vi "SupportedHardware.vi"() -> (3 "Supported Hardware":string[](array[string]))   [LabVIEW 2017, in "McsaFpgaAcquisition.lvlib"]
uses:
  <vilib>/addons/InsightCM/Devices/Shared/Mcsa/McsaFpgaAcquisition/McsaFpgaAcquisition.lvlib
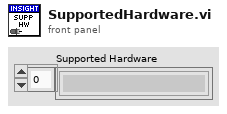
[diagram p1: front panel]
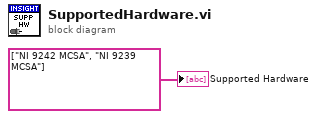
[diagram p0: block diagram]
diagram:
  "Supported Hardware" <- string[] ["NI 9242 MCSA", "NI 9239 MCSA"]
